vi "ClampToggle.vi"(10 "Boolean":bool) -> ()   [LabVIEW 2017]
uses:
  <vilib>/Rock Robotics/WPI/Solenoid/WPI_SolenoidValue.ctl
  <vilib>/Rock Robotics/WPI/Solenoid/WPI_SolenoidSetEnum.vi
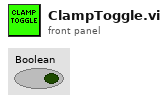
[diagram p1: front panel]
types:
  T1 = typedef "WPI_SolenoidValue.ctl" = enum16{"Off", "On", "Forward", "Reverse"}
  T2 = typedef "WPI_SolenoidDevRef.ctl" = cluster{"DevStatus":errorcluster, "Pneumatics Control Module":u8, "Forward Solenoid Channel":T3, "Reverse Solenoid Channel":T3}
  T3 = typedef "WPI_SolenoidChannel.ctl" = enum8{"Solenoid 0", "Solenoid 1", "Solenoid 2", "Solenoid 3", "Solenoid 4", "Solenoid 5", "Solenoid 6", "Solenoid 7", "Invalid"}
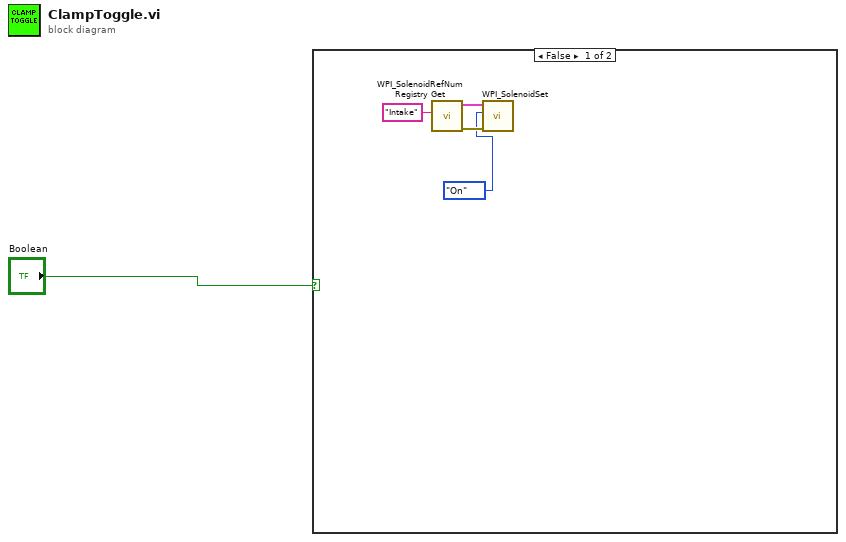
[diagram p0: block diagram]
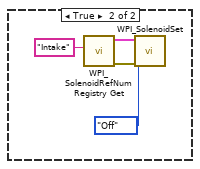
[diagram p2: hidden frame]
diagram:
  n1 = case shown="False" "Boolean" {
    frame False {
      n2 = call <vilib>:"WPI_SolenoidRefNum Registry Get.vi"("refnum name"="Intake") -> ("error out"=w4:errorcluster, "SolenoidDevRef"=w5:T2)  [unwired: 9 in]
      n3 = call-poly <vilib>:"WPI_SolenoidSet.vi"("error in (no error)"=w4, "Value"=WPI_SolenoidValue."On", "SolenoidDevRef"=w5) -> ()  [unwired: 7 in, 2 out]
    }
    frame True {
      n4 = call <vilib>:"WPI_SolenoidRefNum Registry Get.vi"("refnum name"="Intake") -> ("error out"=w9:errorcluster, "SolenoidDevRef"=w8:T2)  [unwired: 9 in]
      n5 = call-poly <vilib>:"WPI_SolenoidSet.vi"("error in (no error)"=w9, "Value"=WPI_SolenoidValue."Off", "SolenoidDevRef"=w8) -> ()  [unwired: 7 in, 2 out]
    }
  }
